vi "ReferenceCurve.vi"(0 "Frequency(GHz)":dbl[](array[numeric])) -> (1 "SGH Gain":dbl[](array[numeric])=[nan, nan, nan, nan, nan, nan, nan, nan, nan, nan, nan, nan, nan, nan, nan, nan, nan, nan, nan, nan, nan, nan, nan, nan, nan, nan, nan, nan, nan, nan, nan, nan, nan, nan, nan, nan, nan, nan, nan, nan, nan, nan, nan, nan, nan, nan, nan, nan, nan, nan, nan, nan, nan, nan, nan, nan, nan, nan, nan, nan, nan, nan, nan, nan, nan, nan, nan, nan, nan, nan, nan, nan, nan, nan, nan, nan, nan, nan, nan, nan, nan, nan, nan, nan, nan, nan, nan, nan, nan, nan, nan, nan, nan, nan, nan, nan, nan, nan, nan, nan, nan, nan, nan, nan, nan, nan, nan, nan, nan, nan, nan, nan, nan, nan, nan, nan, nan, nan, nan, nan, nan, nan, nan, nan, nan, nan, nan, nan, nan, nan, nan, nan, nan, nan, nan, nan, nan, nan, nan, nan, nan, nan, nan, nan, nan, nan, nan, nan, nan, nan, nan, nan, nan, nan, nan, nan, nan, nan, nan, nan, nan, nan, nan, nan, nan, nan, nan, nan, nan, nan, nan, nan, nan, nan, nan, nan, nan, nan, nan, nan, nan, nan, nan, nan, nan, nan, nan, nan, nan, nan, nan, nan, nan, nan, nan, nan, nan, nan, nan, nan, nan, nan, nan, nan, nan, nan, nan, nan, nan, nan, nan, nan, nan, nan, nan, nan, nan, nan, nan, nan, nan, nan, nan, nan, nan, nan, nan, nan, nan, nan, nan, nan, nan, nan, nan, nan, nan, nan, nan, nan, nan, nan, nan, nan, nan, nan, nan, nan, nan, nan, nan, nan, nan, nan, nan, nan, nan, nan, nan, nan, nan, nan, nan, nan, nan, nan, nan, nan, nan, nan, nan, nan, nan, nan, nan, nan, nan, nan, nan, nan, nan, nan, nan, nan, nan, nan, nan, nan, nan, nan, nan, nan, nan, nan, nan, nan, nan, nan, nan, nan, nan, nan, nan, nan, nan, nan, nan, nan, nan, nan, nan, nan, nan, nan, nan, nan, nan, nan, nan, nan, nan, nan, nan, nan, nan, nan, nan, nan, nan, nan, nan, nan, nan, nan, nan, nan, nan, nan, nan, nan, nan, nan, nan, nan, nan, nan, nan, nan, nan, nan, nan, nan, nan, nan, nan, nan, nan, nan, nan, nan, nan, nan, nan, nan, nan, nan, nan, nan, nan, nan, nan, nan, nan, nan, nan, nan, nan, nan, nan, nan, nan, nan, nan, nan, nan, nan, nan, nan, nan, nan, nan, nan, nan, nan, nan, nan, nan, nan, nan, nan, nan], 2 "best fit parameters":dbl[](array[numeric]))   [LabVIEW 2013]
uses:
  <vilib>/gmath/NumericalOptimization/Nonlinear Curve Fit LM formula string.vi
  <vilib>/gmath/NI_Gmath.lvlib
panel:
  in  "initial parameters":dbl[](array[numeric])=[1.0, 1.0, 1.0]
  out "XY Graph":cluster{"X":dbl[], "Best Linear Fit":dbl[]}[](graph)
  in  "GHz":dbl[](array[numeric])=[1.7, 1.9, 2.0, 2.2, 2.3, 2.4]
  in  "dBi":dbl[](array[numeric])=[14.5, 15.3, 15.6, 16.2, 16.5, 16.8]
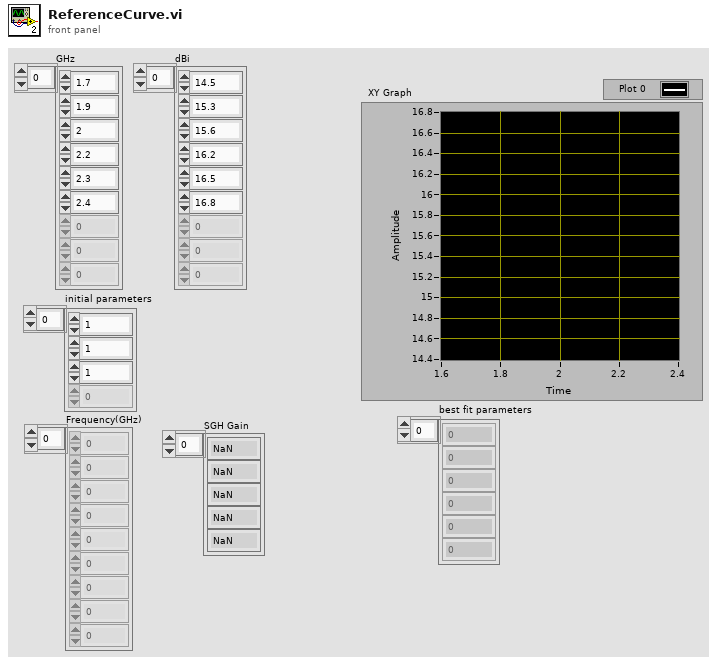
[diagram p1: front panel]
types:
  T1 = cluster{"model":string, "Parameters":string[], "x":string}
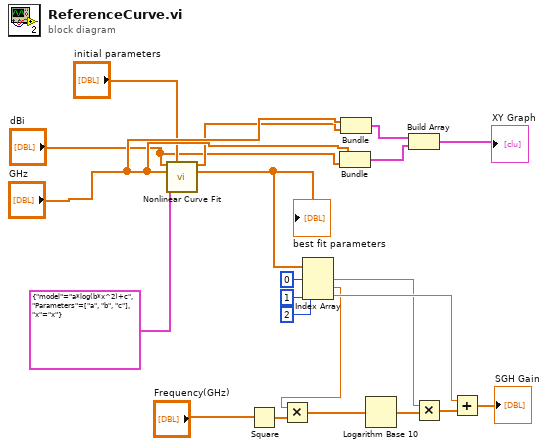
[diagram p0: block diagram]
diagram:
  n1 = call-poly <vilib>:"Nonlinear Curve Fit.vi"("Y"="dBi", "initial parameters"="initial parameters", "X"="GHz", "model description"=T1 {"model"="a*log(b*x^2)+c", "Parameters"=["a", "b", "c"], "x"="x"}) -> ("best nonlinear fit"=w2:dbl[], "best fit parameters"=w8:dbl[])  [unwired: 7 in, 3 out]
  "best fit parameters" <- w8
  n2 = Square(x="Frequency(GHz)") -> (x^2=w13:dbl[])
  n3 = Index Array(array=w8, index #1=0 ("index"), index #2=1 ("index"), index #3=2 ("index")) -> (element #1=w16:dbl, element #2=w14:dbl, element #3=w18:dbl)
  n4 = Multiply(x=w14, y=w13) -> (x*y=w12:dbl[])
  n5 = Bundle("GHz"="GHz", "dBi"="dBi") -> (w6:cluster{"GHz":dbl[], "dBi":dbl[]})  [unwired: 1 in]
  n6 = Bundle("GHz"="GHz", "best nonlinear fit"=w2) -> (w7:cluster{"GHz":dbl[], "best nonlinear fit":dbl[]})  [unwired: 1 in]
  n7 = Logarithm Base 10(1:w12) -> (0:w15:dbl[])
  n8 = Build Array(w7, w6) -> (→"XY Graph":cluster{"GHz":dbl[], "dBi":dbl[]}[])
  n9 = Multiply(x=w16, y=w15) -> (x*y=w17:dbl[])
  n10 = Add(x=w18, y=w17) -> (x+y=→"SGH Gain":dbl[])
